vi "Synthesize By Channel.vi"(6 "last":bool, 8 "error in (no error)":errorcluster, 9 "Repetition":i32, 11 "SigMan in":refnum<class "SignalManager.lvclass">) -> (0 "error out":errorcluster, 2 "Array":dbl[][](array[numeric]), 3 "SigMan out":refnum<class "SignalManager.lvclass">)   [LabVIEW 2020, in "SignalManager.lvclass"]
uses:
  SignalManager.lvclass
  Channel/Channel.lvclass
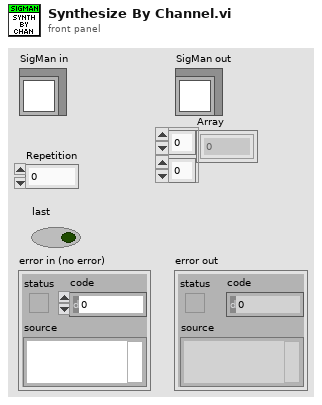
[diagram p1: front panel]
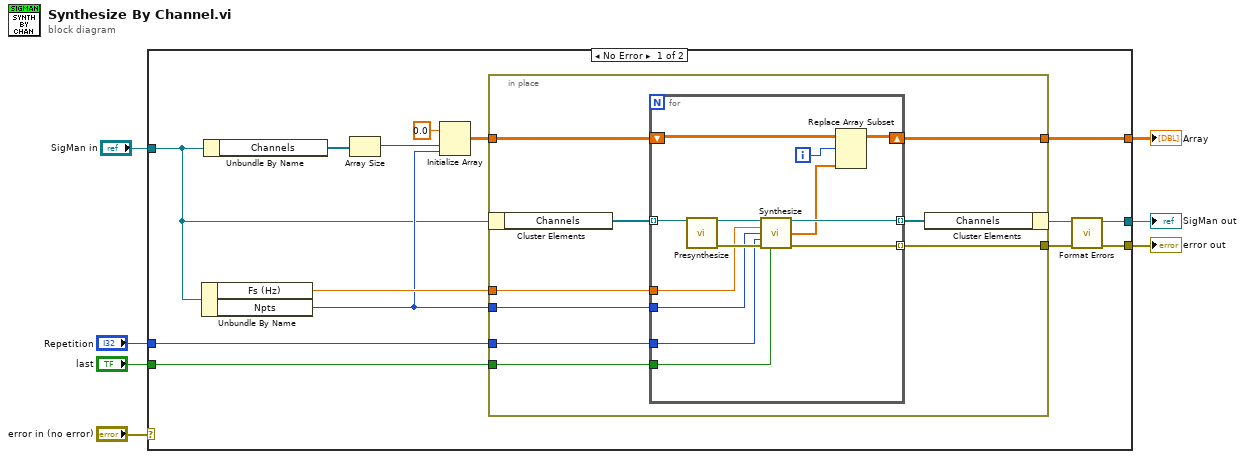
[diagram p0: block diagram]
diagram:
  n1 = case shown="No Error" "error in (no error)" {
    selector: "error in (no error)" -> [_ w45]
    tunnel: [w12 w45] -> w6
    tunnel: [w13 w44] -> w4
    tunnel: "SigMan in" -> [w10 w44]
    tunnel: "Repetition" -> [w18 _]
    tunnel: [w16 _] -> w2
    tunnel: "last" -> [w11 _]
    frame No Error {
      n2 = Unbundle By Name(w10) -> ("Fs (Hz)"=w20:dbl, "Npts"=w19:i32)
      n3 = Unbundle By Name(w10) -> ("Channels"=w9:refnum<class "Channel.lvclass">[])
      n4 = Array Size(array=w9) -> (size(s)=w8:i32)
      n5 = Initialize Array(0.0 ("element"), w8, w19) -> (w17:dbl[][])
      n6 = in-place {
        in-place-border: w20 -> [w29]
        in-place-border: w19 -> [w28]
        in-place-border: w18 -> [w27]
        in-place-border: w17 -> [w26]
        in-place-border: [w24] -> w16
        in-place-border: [w23] -> w14
        in-place-border: w11 -> [w22]
        n7 = in-place-cluster #1(w10) -> ("Channels"=w30:refnum<class "Channel.lvclass">[])
        n8 = for {
          tunnel: w30 -> [w36] mode=indexing
          tunnel: w29 -> [w42]
          tunnel: w28 -> [w41]
          tunnel: w27 -> [w40]
          shift-right: [w37] -> w24
          shift-left: w26 -> [w38]
          tunnel: [w39] -> w25 mode=indexing
          tunnel: [w34] -> w23 mode=indexing
          tunnel: w22 -> [w33]
          i -> [w32]
          n9 = call "Presynthesize.vi"("Channel in"=w36) -> ("Channel out"=w35:refnum<class "Channel.lvclass">, "error out"=w43:errorcluster)  [unwired: 13 in]
          n10 = call "Synthesize.vi"("Channel in"=w35, "Fs (Hz)"=w42, "Npts"=w41, "Repetition"=w40, "error in (no error)"=w43, "last"=w33) -> ("Channel out"=w39:refnum<class "Channel.lvclass">, "Array"=w31:dbl[], "error out"=w34:errorcluster)  [unwired: 6 in, 1 out]
          n11 = Replace Array Subset(array=w38, new element=w31, index (row)=w32) -> (w37:dbl[][])  [unwired: 1 in]
        }
        n12 = in-place-cluster #1("Channels"=w25) -> (w15:refnum<class "SignalManager.lvclass">)
      }
      n13 = call "Format Errors.vi"("error in (no error)"=w14, "SigMan in"=w15) -> ("error out"=w12:errorcluster, "SigMan out"=w13:refnum<class "SignalManager.lvclass">)  [unwired: 8 in]
    }
    frame Error {
    }
  }
  "error out" <- w6
  "SigMan out" <- w4
  "Array" <- w2
